vi "Keypad_1.vi"() -> (2 "Display":string)   [LabVIEW 2015]
panel:
  in  "Dot":bool
  in  "1":bool
  in  "C":bool
  in  "<":bool
  in  "0":bool
  in  "9":bool
  in  "8":bool
  in  "7":bool
  in  "6":bool
  in  "5":bool
  in  "4":bool
  in  "3":bool
  in  "2":bool
  in  "stop":bool
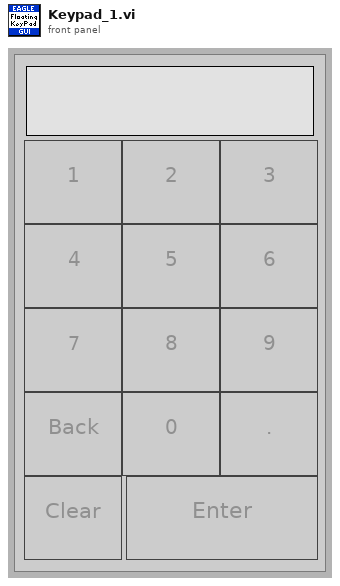
[diagram p1: front panel]
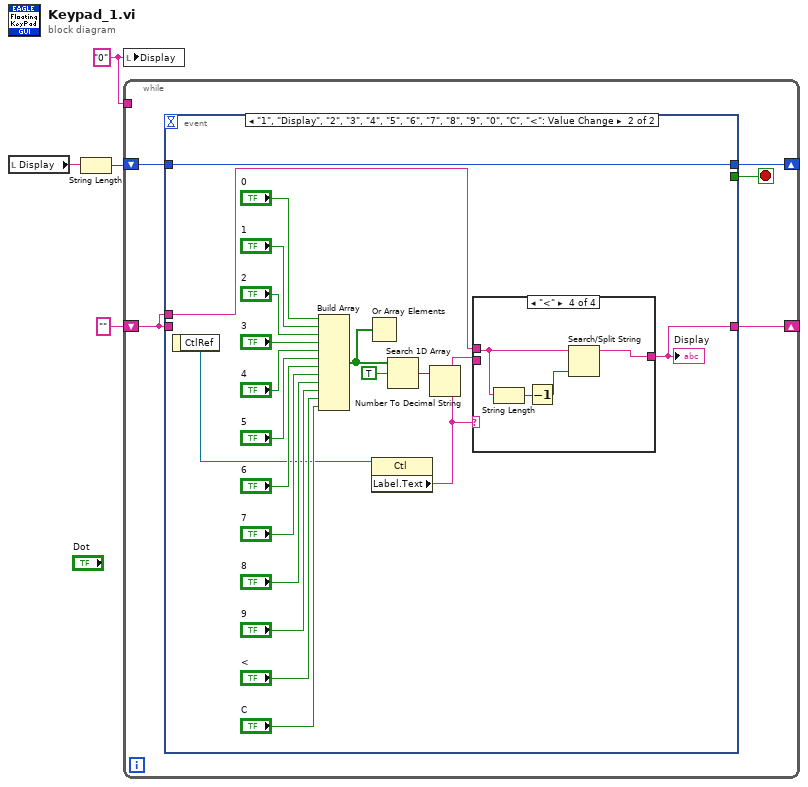
[diagram p0: block diagram]
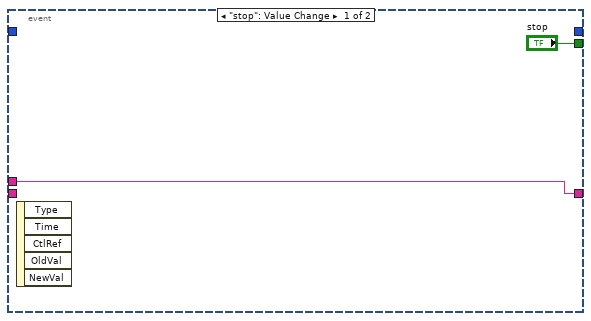
[diagram p2: hidden frame]
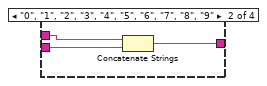
[diagram p4: hidden frame]
diagram:
  w3 = "0" ("String")
  n1 = local read "Display"() -> (w2:string)
  n2 = String Length(string=w2) -> (length=w1:i32)
  n3 = local write "Display"(w3) -> ()
  n4 = while {
    shift-right: [w9] -> _
    shift-left: "" -> [w7]
    tunnel: w3 -> [_]
    shift-right: [w5] -> _
    shift-left: w1 -> [w6]
    stop <- w8 stop-if-true
    n5 = event shown="[1] \"1\", \"Display\", \"2\", \"3\", \"4\", \"5\", \"6\", \"7\", \"8\", \"9\", \"0\", \"C\", \"<\": Value Change" {
      selector: _ -> [_ _]
      dyn-events: _ -> [_ _]
      timeout: _ -> [_ _]
      tunnel: [w11 w17] -> w9
      tunnel: w7 -> [w11 w19]
      tunnel: ["stop" _] -> w8
      tunnel: w7 -> [_ _]
      tunnel: w6 -> [_ w16]
      tunnel: [_ w16] -> w5
      event "stop": Value Change {
        n6 = event-data() -> ()  [unwired: 1 in, 5 out]
      }
      event "1", "Display", "2", "3", "4", "5", "6", "7", "8", "9", "0", "C", "<": Value Change {
        n7 = event-data() -> ("CtlRef"=w13:refnum<vi>)  [unwired: 1 in]
        n8 = Build Array("0", "1", "2", "3", "4", "5", "6", "7", "8", "9", "<", "C") -> (w20:bool[])
        n9 = Or Array Elements(Boolean array=w20) -> ()  [unwired: 1 out]
        n10 = property class="Ctl"(reference=w13) -> ("Label.Text"=w12:string)  [unwired: 1 in, 2 out]
        n11 = Search 1D Array(1D array=w20, element=TRUE) -> (index of element=w18:i32)  [unwired: 1 in]
        n12 = Number To Decimal String(number=w18) -> ()  [unwired: 1 in, 1 out]
        n13 = case shown="\"<\"" w12 {
          tunnel: w12 -> [_ w34 _ _]
          tunnel: w19 -> [w32 w35 _ w39]
          tunnel: [w32 w33 _ w36] -> w17
          frame Default {
          }
          frame "0", "1", "2", "3", "4", "5", "6", "7", "8", "9" {
            n14 = Concatenate Strings(w35, w34) -> (w33:string)
          }
          frame "C" {
          }
          frame "<" {
            n15 = String Length(string=w39) -> (length=w38:i32)
            n16 = Decrement(x=w38) -> (x-1=w37:i32)
            n17 = Search/Split String(string=w39, offset (0)=w37) -> (substring before match=w36:string)  [unwired: 1 in, 2 out]
          }
        }
        "Display" <- w17
      }
    }
  }
